vi "Add VIs to lvlib Virtual Folder.vi"(7 "Virtual Folder Name":string, 8 "error in":errorcluster, 10 "VIs to add":path[](array[path]), 11 "lvlib Path":path) -> (0 "error out":errorcluster)   [LabVIEW 2026, in "NIVS_CDEW_MetaDataObj.lvclass"]
uses:
  NIVS_CDEW_MetaDataObj.lvclass
  NIVS_CDEW_MetaDataObj.lvclass/NIVS_CDEW_MetaDataObj.ctl
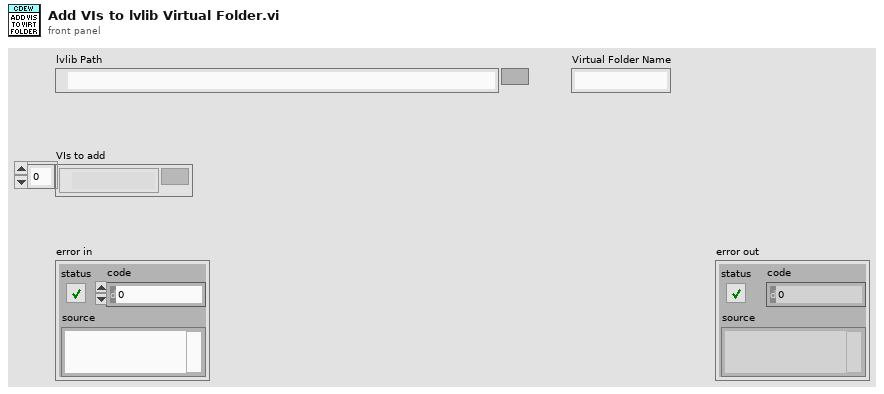
[diagram p1: front panel]
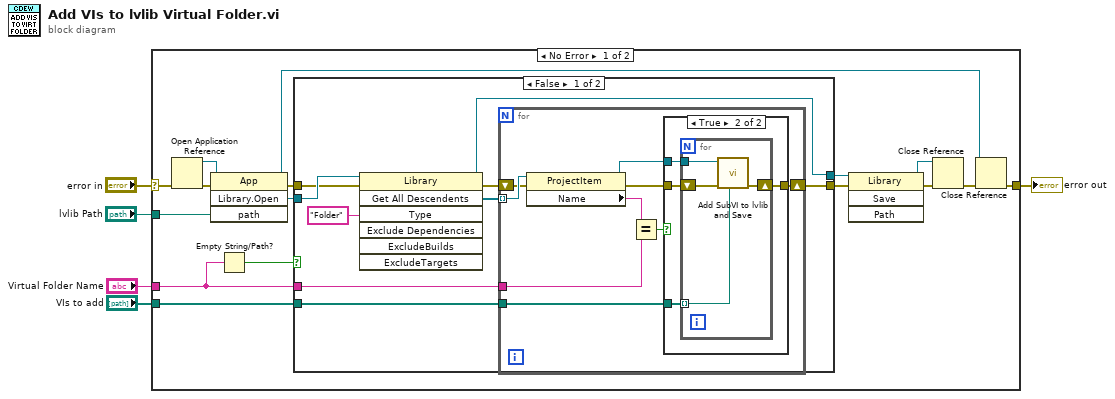
[diagram p0: block diagram]
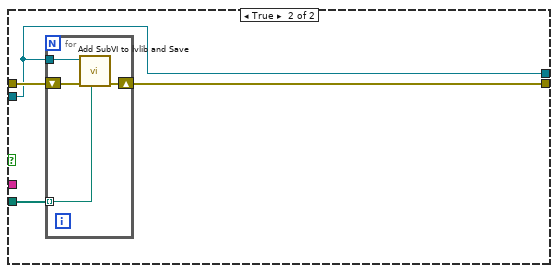
[diagram p3: hidden frame]
diagram:
  n1 = case shown="No Error" "error in" {
    selector: "error in" -> [w17 w57]
    tunnel: "lvlib Path" -> [w14 _]
    tunnel: [w18 w57] -> w4
    tunnel: "Virtual Folder Name" -> [w12 _]
    tunnel: "VIs to add" -> [w13 _]
    frame No Error {
      n2 = Open Application Reference(8:w17) -> (0:w20:errorcluster, 3:w21:refnum<vi>)  [unwired: 3 in]
      n3 = invoke class="App" method="Library.Open"(reference=w21, error in=w20, "path"=w14) -> (reference out=w19:refnum<vi>, error out=w15:errorcluster, "Open Library"=w16:refnum<vi>)  [unwired: 1 in, 1 out]
      n4 = Empty String/Path?(string/path=w12) -> (empty?=w11:bool)
      n5 = case shown="False" w11 {
        tunnel: w16 -> [w30 w49]
        tunnel: w15 -> [w26 w52]
        tunnel: [w23 w51] -> w7
        tunnel: w13 -> [w25 w50]
        tunnel: w12 -> [w24 _]
        tunnel: [w22 w49] -> w6
        frame False {
          n6 = invoke class="Library" method="Get All Descendents"(reference=w30, error in=w26, "Type"="Folder") -> (reference out=w22:refnum<vi>, error out=w27:errorcluster, "All Descendents"=w29:refnum<vi>[])  [unwired: 4 in, 4 out]
          n7 = for {
            tunnel: w29 -> [w39] mode=indexing
            shift-right: [w35] -> w23
            shift-left: w27 -> [w38]
            tunnel: w24 -> [w33]
            tunnel: w25 -> [w31]
            n8 = property class="ProjectItem"(reference=w39, error in=w38) -> (reference out=w36:refnum<vi>, error out=w37:errorcluster, "Name"=w34:string)
            n9 = Equal?(x=w34, y=w33) -> (x = y?=w32:bool)
            n10 = case shown="True" w32 {
              tunnel: w37 -> [w40 w43]
              tunnel: w36 -> [_ w44]
              tunnel: [w40 w42] -> w35
              tunnel: w31 -> [_ w41]
              frame False {
              }
              frame True {
                n11 = for {
                  tunnel: w44 -> [w48]
                  shift-right: [w46] -> w42
                  shift-left: w43 -> [w47]
                  tunnel: w41 -> [w45] mode=indexing
                  n12 = call "Add SubVI to lvlib and Save.vi"("vi path"=w45, "error in"=w47, "ProjectItem"=w48) -> ("error out"=w46:errorcluster)  [unwired: 8 in]
                }
              }
            }
          }
        }
        frame True {
          n13 = for {
            tunnel: w49 -> [w55]
            tunnel: w50 -> [w53] mode=indexing
            shift-right: [w54] -> w51
            shift-left: w52 -> [w56]
            n14 = call "Add SubVI to lvlib and Save.vi"("vi path"=w53, "error in"=w56, "ProjectItem"=w55) -> ("error out"=w54:errorcluster)  [unwired: 8 in]
          }
        }
      }
      n15 = invoke class="Library" method="Save"(reference=w6, error in=w7) -> (reference out=w10:refnum<vi>, error out=w9:errorcluster)  [unwired: 2 in, 2 out]
      n16 = Close Reference(reference=w10, error in (no error)=w9) -> (error out=w8:errorcluster)
      n17 = Close Reference(reference=w19, error in (no error)=w8) -> (error out=w18:errorcluster)
    }
    frame Error {
    }
  }
  "error out" <- w4
